vi "Write AcqType.vi"(8 "error in (no error)":errorcluster, 10 "AcqType":T1(ring), 11 "S4GUI in":refnum<class "S4GUI.lvclass">) -> (0 "error out":errorcluster, 3 "S4GUI out":refnum<class "S4GUI.lvclass">)   [LabVIEW 2018]
uses:
  S4GUI.lvclass
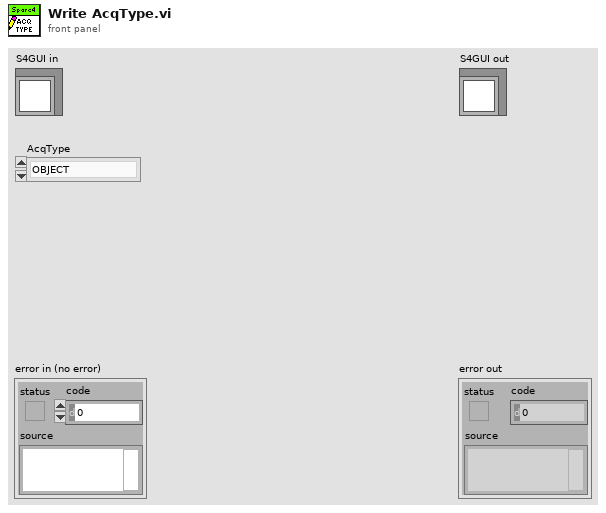
[diagram p1: front panel]
types:
  T1 = enum32{"OBJECT", "DFLAT", "SFLAT", "DARK", "ZERO", "FOCUS"}
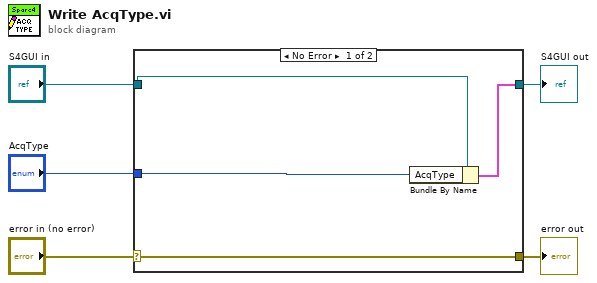
[diagram p0: block diagram]
diagram:
  n1 = case shown="No Error" "error in (no error)" {
    selector: "error in (no error)" -> [w9 w10]
    tunnel: [w9 w10] -> w4
    tunnel: [w7 w11] -> w2
    tunnel: "S4GUI in" -> [w8 w11]
    tunnel: "AcqType" -> [w6 _]
    frame No Error {
      n2 = Bundle By Name(cluster=w8, "AcqType"=w6) -> (w7:cluster{})
    }
    frame Error {
    }
  }
  "error out" <- w4
  "S4GUI out" <- w2
